vi "二進位轉換 (SubVI).vi"(1 "十進位":dbl) -> (0 "二進位":dbl[](array[numeric]))   [LabVIEW 2014]
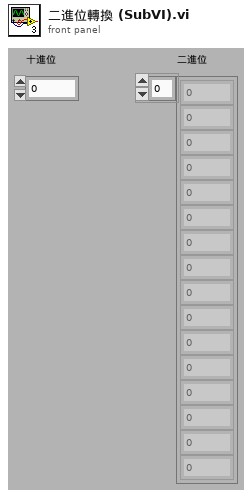
[diagram p1: front panel]
types:
  T1 = cluster{dbl, dbl, dbl, dbl, dbl, dbl, dbl, dbl, dbl, dbl, dbl, dbl, dbl, dbl, dbl, dbl}
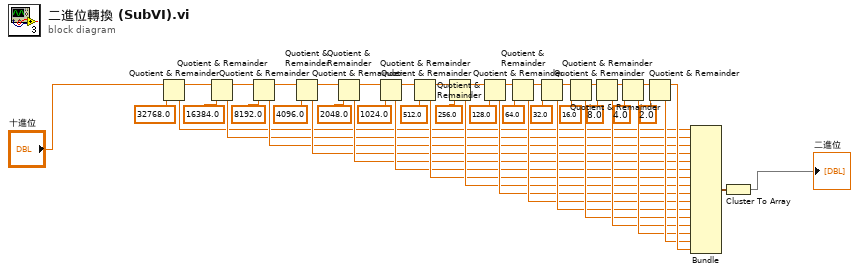
[diagram p0: block diagram]
diagram:
  n1 = Quotient & Remainder(x="十進位", y=32768.0) -> (x-y*floor(x/y)=w5:dbl, floor(x/y)=w13:dbl)
  n2 = Quotient & Remainder(x=w5, y=16384.0) -> (x-y*floor(x/y)=w7:dbl, floor(x/y)=w14:dbl)
  n3 = Quotient & Remainder(x=w7, y=8192.0) -> (x-y*floor(x/y)=w12:dbl, floor(x/y)=w15:dbl)
  n4 = Quotient & Remainder(x=w12, y=4096.0) -> (x-y*floor(x/y)=w10:dbl, floor(x/y)=w17:dbl)
  n5 = Quotient & Remainder(x=w10, y=2048.0) -> (x-y*floor(x/y)=w8:dbl, floor(x/y)=w18:dbl)
  n6 = Quotient & Remainder(x=w8, y=1024.0) -> (x-y*floor(x/y)=w20:dbl, floor(x/y)=w25:dbl)
  n7 = Quotient & Remainder(x=w20, y=512.0) -> (x-y*floor(x/y)=w24:dbl, floor(x/y)=w26:dbl)
  n8 = Quotient & Remainder(x=w24, y=256.0) -> (x-y*floor(x/y)=w21:dbl, floor(x/y)=w27:dbl)
  n9 = Quotient & Remainder(x=w21, y=128.0) -> (x-y*floor(x/y)=w29:dbl, floor(x/y)=w40:dbl)
  n10 = Quotient & Remainder(x=w29, y=64.0) -> (x-y*floor(x/y)=w33:dbl, floor(x/y)=w41:dbl)
  n11 = Quotient & Remainder(x=w33, y=32.0) -> (x-y*floor(x/y)=w30:dbl, floor(x/y)=w42:dbl)
  n12 = Quotient & Remainder(x=w30, y=16.0) -> (x-y*floor(x/y)=w39:dbl, floor(x/y)=w43:dbl)
  n13 = Quotient & Remainder(x=w39, y=8.0) -> (x-y*floor(x/y)=w36:dbl, floor(x/y)=w44:dbl)
  n14 = Quotient & Remainder(x=w36, y=4.0) -> (x-y*floor(x/y)=w34:dbl, floor(x/y)=w45:dbl)
  n15 = Quotient & Remainder(x=w34, y=2.0) -> (x-y*floor(x/y)=w47:dbl, floor(x/y)=w46:dbl)
  n16 = Bundle(w13, w14, w15, w17, w18, w25, w26, w27, w40, w41, w42, w43, w44, w45, w46, w47) -> (w48:T1)  [unwired: 1 in]
  n17 = Cluster To Array(cluster=w48) -> (array=→"二進位":dbl[])
